vi "P18_An_Out.vi"() -> ()   [LabVIEW 2022 SP3]
panel:
  in  "Slide":dbl(slide) scale=0.0..5.0
  in  "stop":bool
  # "P18b_An_Out"
  # "Equipo C\nJairo Issac García López\nRodolfo Durón Hernandez\nRoberto Carlos Herrera Pérez\nSebastián Rodríguez Posada"
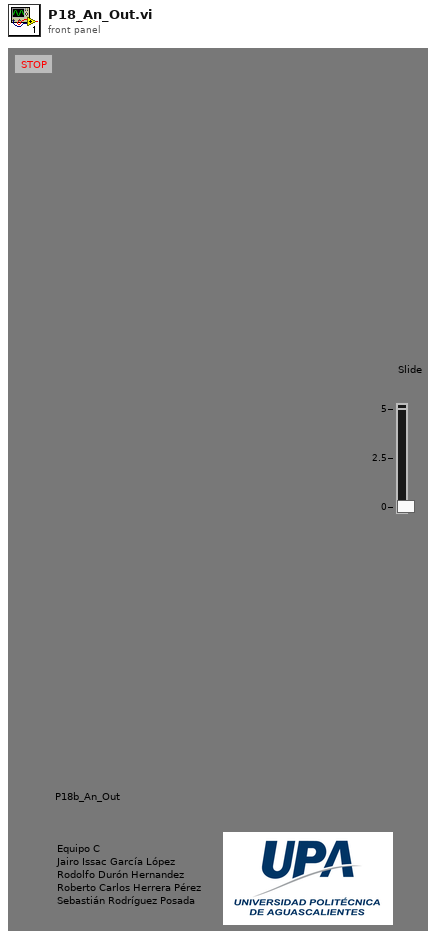
[diagram p1: front panel]
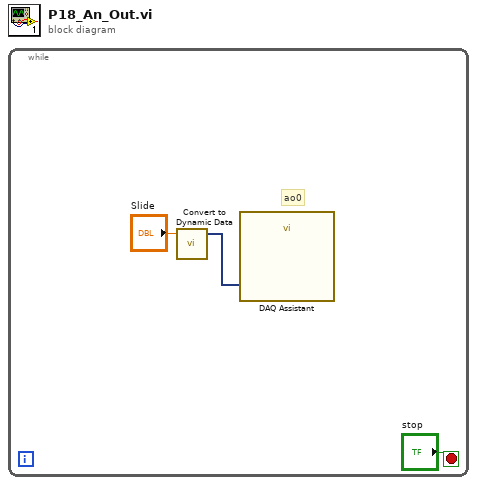
[diagram p0: block diagram]
diagram:
  n1 = while {
    stop <- "stop" stop-if-true
    # "ao0"
    n2 = call "Convert to Dynamic Data"("Double"="Slide") -> ("Dynamic Data Type"=w1:dynamicdata)  [unwired: 3 in]
    n3 = call "DAQ Assistant"("data"=w1) -> ()  [unwired: 17 in, 2 out]
  }
